vi "NominalRangeGLOBAL (1).vi"() -> ()   [LabVIEW 2017]
panel:
  in  "Battery Current":dbl[](array[numeric])=[10.0, 0.0]
  in  "IMU Temperature":dbl[](array[numeric])=[85.0, -20.0]
  in  "Manifold Temperature Range":dbl[](array[numeric])=[60.0, -50.0]
  in  "Tank Temperature Range":dbl[](array[numeric])=[60.0, -50.0]
  in  "Battery Temperature Range":dbl[](array[numeric])=[50.0, -10.0]
  in  "Compact RIO Temperature Range":dbl[](array[numeric])=[80.0, -15.0]
  in  "Battery Voltage":dbl[](array[numeric])=[30.0, 21.0]
  in  "Distance Range":dbl[](array[numeric])=[1609.0, 0.0]
  in  "Piezo Range":dbl[](array[numeric])=[3.4, -0.1]
  in  "Linear Pot Range":dbl[](array[numeric])=[3.4, 0.1]
  in  "Hall Effect Range":dbl[](array[numeric])=[5.1, 0.1]
  in  "Big Tank HPPT":dbl[](array[numeric])=[4000.0, 0.0]
  in  "Baby Tank HPPT":dbl[](array[numeric])=[3500.0, 0.0]
  in  "Low Pressure PT Range":dbl[](array[numeric])=[90.0, 0.0]
  # "Index 0: Upper bound\nIndex 1: Lower bound"
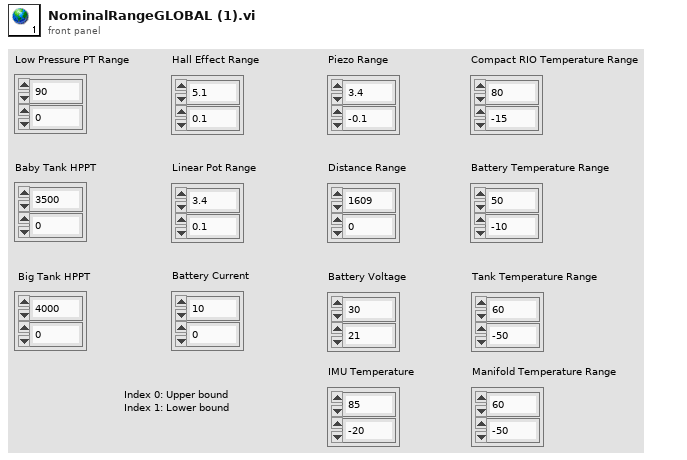
[diagram p1: front panel]
diagram:
